vi "Get Instances Helper.vi"   [LabVIEW 2014, in "LVCOOOP.lvlib" / "Lookup API.lvlib" / "Lookup Service.lvclass"]
doc: "A helper that includes type-casting to the target class."
uses:
  Lookup Service.lvclass
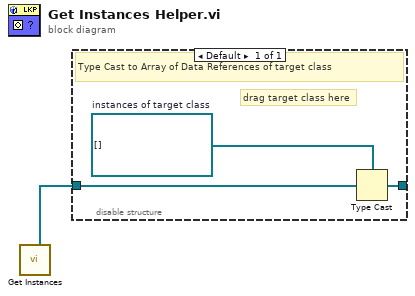
[diagram p0: block diagram]
diagram:
  n1 = call "Get Instances.vi"() -> ("instances"=w1:refnum<data-value>[])  [unwired: 9 in, 2 out]
  n2 = disable-structure shown="Default" {
    disable-tunnel: w1 -> [w4]
    disable-tunnel: [w2] -> _
    frame Enabled {
      w3 = refnum<data-value>[] []  # instances of target class
      # "drag target class here"
      # "Type Cast to Array of Data References of target class"
      n3 = Type Cast(type=w3, x=w4) -> (*(type *) &x=w2:refnum<data-value>[])
    }
  }
